vi "BLTargetsGather.vi"() -> (1 "BL Targets out":T1[](array[typedef]) {"n" min=0.02 max=0.5 step=0.01 format="%.2f"})   [LabVIEW 2022 SP3]
uses:
  BLTarget.ctl
  Globals/Constants_global.vi
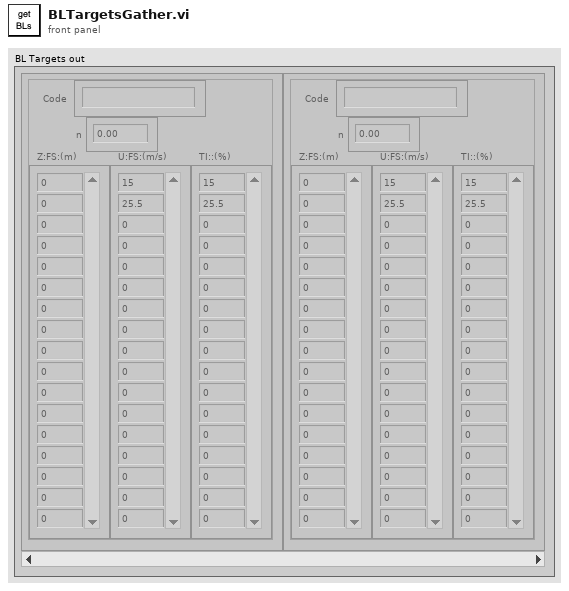
[diagram p1: front panel]
types:
  T1 = typedef "BLTarget.ctl" = cluster{"Code":string, "n":dbl, "Z:FS:(m)":dbl[], "U:FS:(m/s)":dbl[], "TI::(%)":dbl[]}
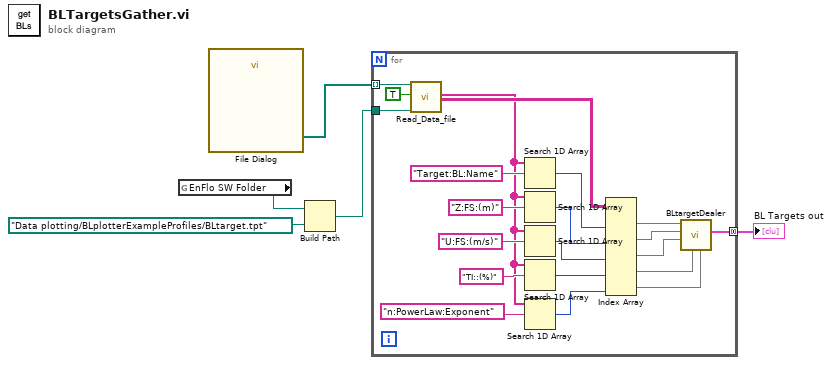
[diagram p0: block diagram]
diagram:
  n1 = global read "Constants_global.vi" "EnFlo SW Folder"() -> (w4:path)
  n2 = call "File Dialog"() -> ("selected paths"=w2:path[])  [unwired: 12 in, 3 out]
  n3 = Build Path(base path=w4, name or relative path=path "Data plotting/BLplotterExampleProfiles/BLtarget.tpt" ("Template File")) -> (appended path=w3:path)
  n4 = for {
    tunnel: w2 -> [w26] mode=indexing
    tunnel: w3 -> [w24]
    tunnel: [w10] -> w1 mode=concatenating
    n5 = call "Read_Data_file.vi"("Results file"=w26, "Delete First Rows?"=TRUE, "Template File"=w24) -> ("Ch names Out"=w7:string[], "Channel Values Out"=w19:string[][])  [unwired: 7 in, 8 out]
    n6 = Search 1D Array(1D array=w7, element="Target:BL:Name") -> (index of element=w18:i32)  [unwired: 1 in]
    n7 = Search 1D Array(1D array=w7, element="Z:FS:(m)") -> (index of element=w17:i32)  [unwired: 1 in]
    n8 = Search 1D Array(1D array=w7, element="U:FS:(m/s)") -> (index of element=w16:i32)  [unwired: 1 in]
    n9 = Search 1D Array(1D array=w7, element="TI::(%)") -> (index of element=w15:i32)  [unwired: 1 in]
    n10 = Search 1D Array(1D array=w7, element="n:PowerLaw:Exponent") -> (index of element=w8:i32)  [unwired: 1 in]
    n11 = Index Array(array=w19, index (col) #1=w18, index (col) #2=w17, index (col) #3=w16, index (col) #4=w15, index (col) #5=w8) -> (element #1=w14:string[], element #2=w13:string[], element #3=w12:string[], element #4=w11:string[], element #5=w6:string[])  [unwired: 5 in]
    n12 = call "BLtargetDealer.vi"("n"=w6, "TI"=w11, "U"=w12, "Z"=w13, "Name"=w14) -> ("BLtargets"=w10:T1[])  [unwired: 6 in]
  }
  "BL Targets out" <- w1
